vi "save_to_spreadsheet_activity25.vi"() -> ()   [LabVIEW 2025]
uses:
  <vilib>/Utility/file.llb/Write Delimited Spreadsheet (DBL).vi
panel:
  out "Waveform array":dbl[](array[numeric])
  out "Waveform Graph":cluster{dbl[]}[](graph)
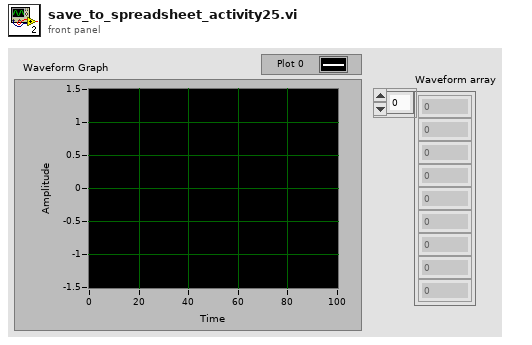
[diagram p1: front panel]
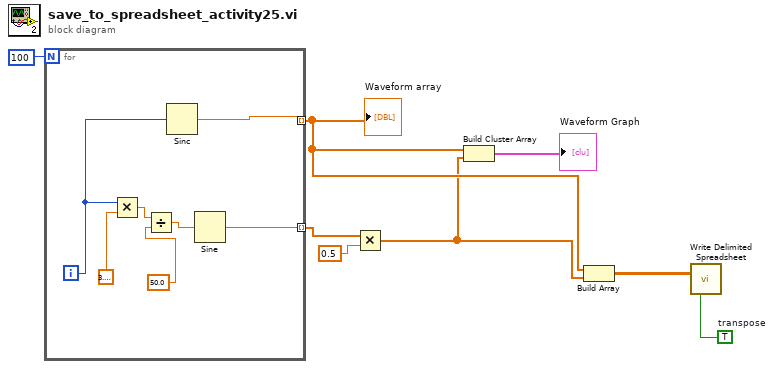
[diagram p0: block diagram]
diagram:
  w5 = TRUE  # transpose
  n1 = for {
    N: 100 -> [_]
    tunnel: [w15] -> w7 mode=indexing
    tunnel: [w10] -> w3 mode=indexing
    i -> [w9]
    n2 = Multiply(x=w9, y=3.141592653589793) -> (x*y=w13:dbl)
    n3 = Divide(x=w13, y=50.0) -> (x/y=w11:dbl)
    n4 = Sinc(1:w9) -> (0:w10:dbl)
    n5 = Sine(x=w11) -> (sin(x)=w15:dbl)
  }
  "Waveform array" <- w3
  n6 = Multiply(x=w7, y=0.5) -> (x*y=w2:dbl[])
  n7 = Build Cluster Array(w3, w2) -> (→"Waveform Graph":cluster{dbl[]}[])
  n8 = Build Array(w3, w2) -> (w1:dbl[][])
  n9 = call-poly <vilib>:"Write Delimited Spreadsheet.vi"("2D data"=w1, "transpose? (no:F)"=w5) -> ()  [unwired: 12 in, 2 out]
